vi "initiate.vi"(0 "reference in":refnum<class "GUI Controller.lvclass">, 5 "error in (no error)":errorcluster) -> (14 "reference out":refnum<class "GUI Controller.lvclass">, 19 "error out":errorcluster)   [LabVIEW 2015, in "GUI Controller.lvclass"]
uses:
  GUI Controller.lvclass
  Project Panels_class/Project Panels.lvclass
  SYS/Items Controller_llb/Items Controller.lvclass
  SYS/Notification Controller_class/Notification Controller.lvclass
  SYS/PartsTracking Controller_class/PartsTracking Controller.lvclass
  SYS/File Controller_llb/File Controller.lvclass
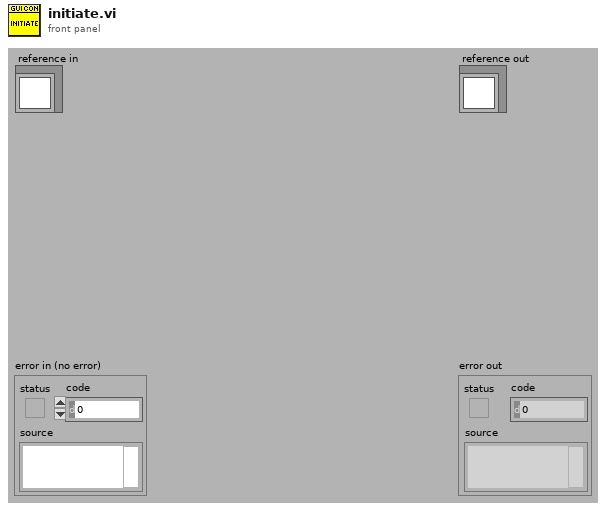
[diagram p1: front panel]
types:
  T1 = typedef "GUI Controller.lvclass/ObjectAttributesRef.ctl" = refnum<data-value>
  T2 = typedef "GUI Controller.lvclass/ObjectAttributes.ctl" = cluster{"MyAttribute":dbl, "state":T3, "project_panels_ref":refnum<class "Project Panels.lvclass">, "items_controller_ref":refnum<class "Items Controller.lvclass">, "notification_controller_ref":refnum<class "Notification Controller.lvclass">, "partstracking_controller_ref":refnum<class "PartsTracking Controller.lvclass">, "file_controller_ref":refnum<class "File Controller.lvclass">, "low_resolution?":bool}
  T3 = typedef "GUI Controller.lvclass/state.ctl" = enum16{"initiate", "checkNotificationItems", "checkNotificationTracking", "operate", "updateFromFile", "stop"}
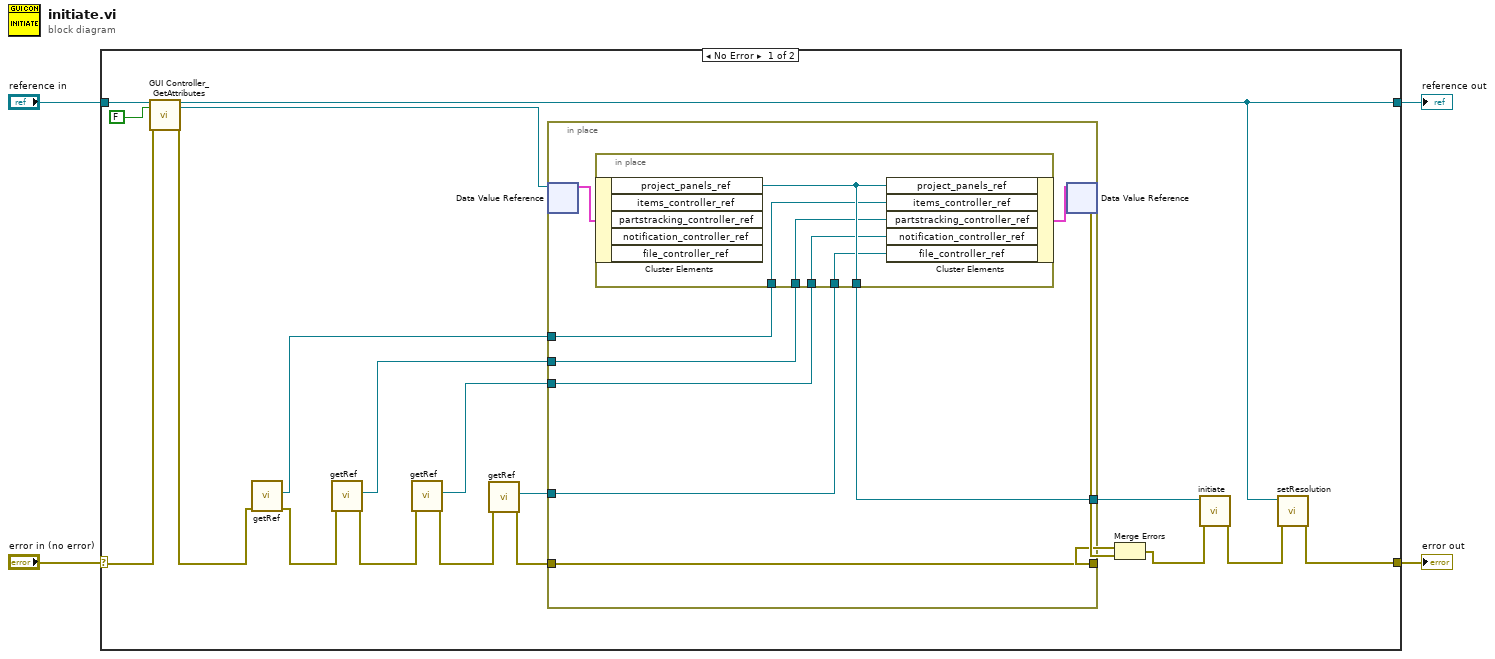
[diagram p0: block diagram]
diagram:
  n1 = case shown="No Error" "error in (no error)" {
    selector: "error in (no error)" -> [w20 w39]
    tunnel: [w5 w39] -> w3
    tunnel: [w7 w38] -> w1
    tunnel: "reference in" -> [w22 w38]
    frame No Error {
      n2 = call "GUI Controller_GetAttributes.vi"("reference in"=w22, "return data? (T)"=FALSE, "error in (no error)"=w20) -> ("reference out"=w7:refnum<class "GUI Controller.lvclass">, "attributes ref"=w19:T1, "error out"=w16:errorcluster)  [unwired: 13 in, 1 out]
      n3 = call "getRef.vi"("error in (no error)"=w16) -> ("error out"=w14:errorcluster, "items_controller_ref"=w15:refnum<class "Items Controller.lvclass">)  [unwired: 9 in]
      n4 = call "getRef.vi"("error in (no error)"=w14) -> ("error out"=w12:errorcluster, "partstracking_controller_ref"=w13:refnum<class "PartsTracking Controller.lvclass">)  [unwired: 9 in]
      n5 = call "getRef.vi"("error in (no error)"=w12) -> ("error out"=w10:errorcluster, "notification_controller_ref"=w11:refnum<class "Notification Controller.lvclass">)  [unwired: 9 in]
      n6 = call "getRef.vi"("error in (no error)"=w10) -> ("error out"=w9:errorcluster, "File Controller_ref"=w8:refnum<class "File Controller.lvclass">)  [unwired: 9 in]
      n7 = in-place {
        in-place-border: w9 -> [w30]
        in-place-border: [w30] -> w23
        in-place-border: [w29] -> w18
        in-place-border: w15 -> [w28]
        in-place-border: w13 -> [w27]
        in-place-border: w11 -> [w26]
        in-place-border: w8 -> [w25]
        n8 = in-place-dvr #1(w19) -> (w31:T2)  [unwired: 1 out]
        n9 = in-place {
          in-place-border: [w37] -> w29
          in-place-border: w28 -> [w36]
          in-place-border: w27 -> [w35]
          in-place-border: w26 -> [w34]
          in-place-border: w25 -> [w33]
          n10 = in-place-cluster #2(w31) -> ("project_panels_ref"=w37:refnum<class "Project Panels.lvclass">)  [unwired: 4 out]
          n11 = in-place-cluster #2("project_panels_ref"=w37, "items_controller_ref"=w36, "partstracking_controller_ref"=w35, "notification_controller_ref"=w34, "file_controller_ref"=w33) -> (w32:T2)
        }
        n12 = in-place-dvr #1(w32) -> (w24:errorcluster)  [unwired: 1 out]
      }
      n13 = Merge Errors(w23, w24) -> (w17:errorcluster)
      n14 = call "initiate.vi"("error in (no error)"=w17, "reference in"=w18) -> ("error out"=w6:errorcluster)  [unwired: 8 in, 1 out]
      n15 = call "setResolution.vi"("error in (no error)"=w6, "reference in"=w7) -> ("error out"=w5:errorcluster)  [unwired: 8 in, 1 out]
    }
    frame Error {
    }
  }
  "error out" <- w3
  "reference out" <- w1
